vi "Get Operating Mode.vi"(8 "error in (no error)":errorcluster, 11 "BNO055 in":refnum<class "BNO055.lvclass">) -> (0 "error out":errorcluster, 2 "Operating Mode":T1, 3 "BNO055 out":refnum<class "BNO055.lvclass">)   [LabVIEW 2020, in "BNO055.lvlib" / "BNO055.lvclass"]
uses:
  BNO055.lvclass
  Operating Mode.ctl
  BNO055.lvclass/BNO055.ctl
  <vilib>/MakerHub/LINX/LMH-LINX.lvlib
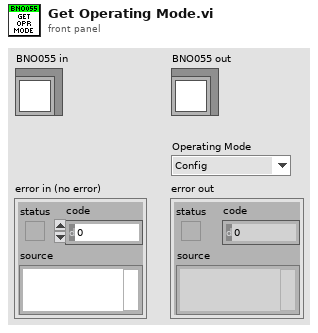
[diagram p1: front panel]
types:
  T1 = typedef "BNO055.lvlib/BNO055.lvclass/Operating Mode.ctl" = enum8{"Config", "Acc Only", "Mag Only", "Gyr Only", "Acc Mag", "Acc Gyr", "Mag Gyr", "AccMagGyr", "IMU", "Compass", "Mag4Gyr", "NDOF FMC Off", "NDOF"}
  T2 = typedef "LMH-LINX.lvlib/LINX Ref.ctl" = cluster{"IO":T3, "Interface":T4, "LINX Device Config":T5}
  T3 = typedef "LMH-LINX.lvlib/Platform.ctl" = enum16{"Remote", "Local"}
  T4 = typedef "LMH-LINX.lvlib/Interface.ctl" = enum16{"Serial", "TCP"}
  T5 = typedef "LMH-LINX.lvlib/Device.lvlib/LINX Device Config.ctl" = cluster{"Interface":T4, "COM Port":refnum<visa-resource-name>, "TCP Configuration":T6, "Device Family":u8, "Device ID":u8, "Device Name":string, "TCP Ref":refnum<k5>, "Channels":T7}
  T6 = typedef "LMH-LINX.lvlib/Device.lvlib/TCP Config.ctl" = cluster{"IP Address":string, "Port":u16}
  T7 = typedef "LMH-LINX.lvlib/Channels.ctl" = cluster{"DI":u8[], "DO":u8[], "AI":u8[], "AO":u8[], "PWM":u8[], "QE":u8[], "UART":u8[], "I2C 2":u8[], "SPI":u8[], "CAN":u8[], "Servo":u8[], "AI Ref (V)":dbl, "AI Resolution (Bits)":u8, "AO Ref (V)":dbl, "AO Resolution (Bits)":u8}
  T8 = typedef "BNO055.lvlib/BNO055.lvclass/Address.ctl" = u8
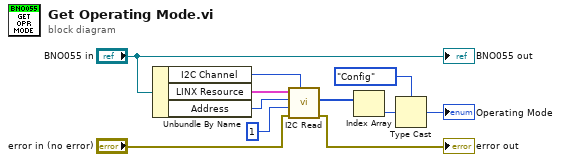
[diagram p0: block diagram]
diagram:
  n1 = Unbundle By Name("BNO055 in") -> ("I2C Channel"=w9:u8, "LINX Resource"=w10:T2, "Address"=w8:T8)
  n2 = call <vilib>:"I2C Read.vi"("I2C Channel"=w9, "Error In"="error in (no error)", "Bytes To Read"=u8 1, "I2C Slave Address (0)"=w8, "LINX Resource"=w10) -> ("Error Out"=→"error out":errorcluster, "Data"=w6:u8[])  [unwired: 4 in, 1 out]
  n3 = Index Array(array=w6) -> (element=w5:u8)  [unwired: 1 in]
  n4 = Type Cast(type=Operating_Mode."Config" ("Operating Mode"), x=w5) -> (*(type *) &x=→"Operating Mode":T1)
  "BNO055 out" <- "BNO055 in"
